vi "analysis.vi"() -> ()   [LabVIEW 2015]
doc: "Program analyzes data files for both constant radioactive decay counting and shor-lived decay experiments."
uses:
  <vilib>/Utility/file.llb/Read Delimited Spreadsheet (DBL).vi
  <vilib>/imath/engines/lvmath2/RunTimeEngine/Managers/WorkSpace/UID Generator.vi
  <vilib>/imath/engines/lvmath2/RunTimeEngine/RunTimeType/NIMS_RunTimeType_From StrictType (excl LVString).vi
  <instcachedir>/0/NIMS_RunTimeType_From StrictType (excl LVString)_EB1C38A9BC5048DA9ABDA8F781E54D21.lvgen/NIMS_RunTimeType_From StrictType (excl LVString)_EB1C38A9BC5048DA9ABDA8F781E54D21_000.vi
  <vilib>/imath/engines/lvmath2/RunTimeEngine/LocalVariableDefStatement/MC_LocalVariableDefStatement_Display.vi
  <vilib>/imath/engines/lvmath2/RunTimeEngine/Managers/SymbolTable/Clear UID.vi
  <vilib>/imath/engines/lvmath2/RunTimeEngine/NodeEndStatement/NIMS_NodeEndStatement_Output.vi
  <instcachedir>/0/NIMS_NodeEndStatement_Output_53EC0D466D134D7ABD903AC30B43404B.lvgen/NIMS_NodeEndStatement_Output_53EC0D466D134D7ABD903AC30B43404B_001.vi
  <vilib>/imath/engines/lvmath2/RunTimeEngine/ErrorHandling/NIMS_Finalize Error.vi
  <vilib>/Analysis/NI_AALBase.lvlib
  <vilib>/Analysis/NI_AALPro.lvlib
  <vilib>/imath/engines/lvmath2/RunTimeEngine/Managers/SymbolTable/NIMS_WorkSpace.lvlib
panel:
  out "Decay Time (s)":dbl=106.21083077427976
  out "Counting Statistics":T1(graph)={"X Values"=[13.5, 14.5, 15.5, 16.5, 17.5, 18.5, 19.5, 20.5, 21.5, 22.5, 23.5, 24.5, 25.5, 26.5, 27.5, 28.5, 29.5, 30.5, 31.5, 32.5, 33.5, 34.5, 35.5], "Histogram: h(x)"=[4, 1, 4, 6, 8, 9, 10, 9, 17, 13, 12, 13, 8, 13, 15, 8, 9, 4, 4, 1, 3, 3, 6]}
  out "Decay Curve":cluster{dbl[], "Best Exponential Fit":dbl[]}[](graph)=[{[1.0, 2.0, 3.0, 4.0, 5.0, 6.0, 7.0, 8.0, 9.0, 10.0, 11.0, 12.0, 13.0, 14.0, 15.0, 16.0, 17.0, 18.0, 19.0, 20.0, 21.0, 22.0, 23.0, 24.0, 25.0, 26.0, 27.0, 28.0, 29.0, 30.0, 31.0, 32.0, 33.0, 34.0, 35.0, 36.0, 37.0, 38.0, 39.0, 40.0, 41.0, 42.0, 43.0, 44.0, 45.0, 46.0, 47.0, 48.0, 49.0, 50.0, 51.0, 52.0, 53.0, 54.0, 55.0, 56.0, 57.0, 58.0, 59.0, 60.0, 61.0, 62.0, 63.0, 64.0, 65.0, 66.0, 67.0, 68.0, 69.0, 70.0, 71.0, 72.0, 73.0, 74.0, 75.0, 76.0, 77.0, 78.0, 79.0, 80.0, 81.0, 82.0, 83.0, 84.0, 85.0, 86.0, 87.0, 88.0, 89.0, 90.0, 91.0, 92.0, 93.0, 94.0, 95.0, 96.0, 97.0, 98.0, 99.0, 100.0, 101.0, 102.0, 103.0, 104.0, 105.0, 106.0, 107.0, 108.0, 109.0, 110.0, 111.0, 112.0, 113.0, 114.0, 115.0, 116.0, 117.0, 118.0, 119.0, 120.0, 121.0, 122.0, 123.0, 124.0, 125.0, 126.0, 127.0, 128.0, 129.0, 130.0, 131.0, 132.0, 133.0, 134.0, 135.0, 136.0, 137.0, 138.0, 139.0, 140.0, 141.0, 142.0, 143.0, 144.0, 145.0, 146.0, 147.0, 148.0, 149.0, 150.0, 151.0, 152.0, 153.0, 154.0, 155.0, 156.0, 157.0, 158.0, 159.0, 160.0, 161.0, 162.0, 163.0, 164.0, 165.0, 166.0, 167.0, 168.0, 169.0, 170.0, 171.0, 172.0, 173.0, 174.0, 175.0, 176.0, 177.0, 178.0, 179.0, 180.0, 181.0, 182.0, 183.0, 184.0, 185.0, 186.0, 187.0, 188.0, 189.0, 190.0, 191.0, 192.0, 193.0, 194.0, 195.0, 196.0, 197.0, 198.0, 199.0, 200.0, 201.0, 202.0, 203.0, 204.0, 205.0, 206.0, 207.0, 208.0, 209.0, 210.0, 211.0, 212.0, 213.0, 214.0, 215.0, 216.0, 217.0, 218.0, 219.0, 220.0, 221.0, 222.0, 223.0, 224.0, 225.0, 226.0, 227.0, 228.0, 229.0, 230.0, 231.0, 232.0, 233.0, 234.0, 235.0, 236.0, 237.0, 238.0, 239.0, 240.0, 241.0, 242.0, 243.0, 244.0, 245.0, 246.0, 247.0, 248.0, 249.0, 250.0, 251.0, 252.0, 253.0, 254.0, 255.0, 256.0, 257.0, 258.0, 259.0, 260.0, 261.0, 262.0, 263.0, 264.0, 265.0, 266.0, 267.0, 268.0, 269.0, 270.0, 271.0, 272.0, 273.0, 274.0, 275.0, 276.0, 277.0, 278.0, 279.0, 280.0, 281.0, 282.0, 283.0, 284.0, 285.0, 286.0, 287.0, 288.0, 289.0, 290.0, 291.0, 292.0, 293.0, 294.0, 295.0, 296.0, 297.0, 298.0, 299.0, 300.0, 301.0, 302.0, 303.0, 304.0, 305.0, 306.0, 307.0, 308.0, 309.0, 310.0, 311.0, 312.0, 313.0, 314.0, 315.0, 316.0, 317.0, 318.0, 319.0, 320.0, 321.0, 322.0, 323.0, 324.0, 325.0, 326.0, 327.0, 328.0, 329.0, 330.0], "Best Exponential Fit"=[80.0, 70.0, 60.0, 68.0, 62.0, 64.0, 57.0, 55.0, 60.0, 67.0, 62.0, 57.0, 54.0, 53.0, 54.0, 49.0, 58.0, 50.0, 44.0, 55.0, 51.0, 60.0, 51.0, 53.0, 45.0, 56.0, 49.0, 39.0, 50.0, 48.0, 53.0, 55.0, 44.0, 45.0, 36.0, 29.0, 36.0, 53.0, 41.0, 38.0, 34.0, 42.0, 50.0, 43.0, 36.0, 42.0, 43.0, 66.0, 32.0, 38.0, 41.0, 36.0, 38.0, 33.0, 33.0, 31.0, 37.0, 34.0, 33.0, 34.0, 33.0, 39.0, 37.0, 19.0, 35.0, 42.0, 35.0, 34.0, 26.0, 32.0, 35.0, 37.0, 34.0, 23.0, 21.0, 25.0, 27.0, 27.0, 30.0, 27.0, 25.0, 34.0, 26.0, 26.0, 25.0, 30.0, 32.0, 27.0, 28.0, 21.0, 29.0, 33.0, 37.0, 27.0, 27.0, 28.0, 25.0, 17.0, 18.0, 14.0, 29.0, 27.0, 27.0, 17.0, 18.0, 25.0, 24.0, 15.0, 21.0, 27.0, 24.0, 18.0, 24.0, 21.0, 16.0, 22.0, 16.0, 19.0, 18.0, 32.0, 21.0, 17.0, 25.0, 17.0, 23.0, 23.0, 17.0, 16.0, 10.0, 17.0, 23.0, 21.0, 26.0, 13.0, 16.0, 15.0, 12.0, 22.0, 21.0, 15.0, 20.0, 17.0, 16.0, 15.0, 21.0, 15.0, 13.0, 20.0, 25.0, 15.0, 14.0, 11.0, 16.0, 20.0, 13.0, 17.0, 15.0, 26.0, 10.0, 12.0, 17.0, 20.0, 13.0, 12.0, 12.0, 13.0, 16.0, 12.0, 11.0, 10.0, 11.0, 13.0, 13.0, 23.0, 10.0, 14.0, 12.0, 6.0, 9.0, 13.0, 10.0, 17.0, 8.0, 8.0, 12.0, 9.0, 10.0, 15.0, 9.0, 14.0, 9.0, 15.0, 11.0, 11.0, 9.0, 21.0, 11.0, 12.0, 8.0, 11.0, 10.0, 9.0, 12.0, 13.0, 11.0, 11.0, 10.0, 9.0, 13.0, 8.0, 11.0, 6.0, 13.0, 8.0, 11.0, 15.0, 11.0, 9.0, 10.0, 8.0, 9.0, 4.0, 6.0, 7.0, 4.0, 5.0, 9.0, 7.0, 7.0, 12.0, 7.0, 6.0, 9.0, 7.0, 7.0, 8.0, 10.0, 6.0, 7.0, 4.0, 7.0, 3.0, 7.0, 2.0, 11.0, 6.0, 9.0, 7.0, 10.0, 13.0, 3.0, 11.0, 7.0, 6.0, 6.0, 6.0, 3.0, 6.0, 4.0, 6.0, 10.0, 9.0, 8.0, 5.0, 6.0, 7.0, 6.0, 3.0, 7.0, 6.0, 4.0, 2.0, 3.0, 3.0, 5.0, 6.0, 3.0, 5.0, 6.0, 8.0, 8.0, 11.0, 6.0, 3.0, 6.0, 4.0, 7.0, 1.0, 2.0, 1.0, 4.0, 2.0, 4.0, 1.0, 7.0, 2.0, 0.0, 4.0, 4.0, 5.0, 4.0, 1.0, 3.0, 2.0, 8.0, 3.0, 4.0, 3.0, 4.0, 7.0, 5.0, 5.0, 2.0, 4.0, 2.0, 7.0, 5.0, 3.0, 2.0, 4.0, 2.0, 3.0, 4.0, 0.0, 3.0, 3.0, 4.0, 4.0, 5.0, 5.0]}, {[1.0, 2.0, 3.0, 4.0, 5.0, 6.0, 7.0, 8.0, 9.0, 10.0, 11.0, 12.0, 13.0, 14.0, 15.0, 16.0, 17.0, 18.0, 19.0, 20.0, 21.0, 22.0, 23.0, 24.0, 25.0, 26.0, 27.0, 28.0, 29.0, 30.0, 31.0, 32.0, 33.0, 34.0, 35.0, 36.0, 37.0, 38.0, 39.0, 40.0, 41.0, 42.0, 43.0, 44.0, 45.0, 46.0, 47.0, 48.0, 49.0, 50.0, 51.0, 52.0, 53.0, 54.0, 55.0, 56.0, 57.0, 58.0, 59.0, 60.0, 61.0, 62.0, 63.0, 64.0, 65.0, 66.0, 67.0, 68.0, 69.0, 70.0, 71.0, 72.0, 73.0, 74.0, 75.0, 76.0, 77.0, 78.0, 79.0, 80.0, 81.0, 82.0, 83.0, 84.0, 85.0, 86.0, 87.0, 88.0, 89.0, 90.0, 91.0, 92.0, 93.0, 94.0, 95.0, 96.0, 97.0, 98.0, 99.0, 100.0, 101.0, 102.0, 103.0, 104.0, 105.0, 106.0, 107.0, 108.0, 109.0, 110.0, 111.0, 112.0, 113.0, 114.0, 115.0, 116.0, 117.0, 118.0, 119.0, 120.0, 121.0, 122.0, 123.0, 124.0, 125.0, 126.0, 127.0, 128.0, 129.0, 130.0, 131.0, 132.0, 133.0, 134.0, 135.0, 136.0, 137.0, 138.0, 139.0, 140.0, 141.0, 142.0, 143.0, 144.0, 145.0, 146.0, 147.0, 148.0, 149.0, 150.0, 151.0, 152.0, 153.0, 154.0, 155.0, 156.0, 157.0, 158.0, 159.0, 160.0, 161.0, 162.0, 163.0, 164.0, 165.0, 166.0, 167.0, 168.0, 169.0, 170.0, 171.0, 172.0, 173.0, 174.0, 175.0, 176.0, 177.0, 178.0, 179.0, 180.0, 181.0, 182.0, 183.0, 184.0, 185.0, 186.0, 187.0, 188.0, 189.0, 190.0, 191.0, 192.0, 193.0, 194.0, 195.0, 196.0, 197.0, 198.0, 199.0, 200.0, 201.0, 202.0, 203.0, 204.0, 205.0, 206.0, 207.0, 208.0, 209.0, 210.0, 211.0, 212.0, 213.0, 214.0, 215.0, 216.0, 217.0, 218.0, 219.0, 220.0, 221.0, 222.0, 223.0, 224.0, 225.0, 226.0, 227.0, 228.0, 229.0, 230.0, 231.0, 232.0, 233.0, 234.0, 235.0, 236.0, 237.0, 238.0, 239.0, 240.0, 241.0, 242.0, 243.0, 244.0, 245.0, 246.0, 247.0, 248.0, 249.0, 250.0, 251.0, 252.0, 253.0, 254.0, 255.0, 256.0, 257.0, 258.0, 259.0, 260.0, 261.0, 262.0, 263.0, 264.0, 265.0, 266.0, 267.0, 268.0, 269.0, 270.0, 271.0, 272.0, 273.0, 274.0, 275.0, 276.0, 277.0, 278.0, 279.0, 280.0, 281.0, 282.0, 283.0, 284.0, 285.0, 286.0, 287.0, 288.0, 289.0, 290.0, 291.0, 292.0, 293.0, 294.0, 295.0, 296.0, 297.0, 298.0, 299.0, 300.0, 301.0, 302.0, 303.0, 304.0, 305.0, 306.0, 307.0, 308.0, 309.0, 310.0, 311.0, 312.0, 313.0, 314.0, 315.0, 316.0, 317.0, 318.0, 319.0, 320.0, 321.0, 322.0, 323.0, 324.0, 325.0, 326.0, 327.0, 328.0, 329.0, 330.0], "Best Exponential Fit"=[62.77238848490245, 62.184145225125434, 61.60141442299143, 61.024144420978196, 60.4522840456488, 59.885782603115175, 59.324589874544294, 58.768656111706356, 58.217932032564796, 57.6723688169075, 57.13191810201907, 56.59653197839359, 56.06616298548755, 55.54076410751265, 55.02028876926792, 54.504690832010986, 53.99392458936799, 53.48794476328183, 52.98670649999839, 52.490165366090395, 51.99827734451846, 51.51099883072915, 51.02828662878951, 50.55009794755788, 50.07639039689059, 49.60712198388416, 49.14225110915277, 48.681736563140525, 48.22553752246845, 47.773613546315495, 47.325924572833614, 46.882430915596395, 46.443093260080964, 46.007872660182834, 45.57673053476346, 45.149628664230114, 44.72652918714783, 44.30739459688307, 43.89218773827891, 43.48087180436125, 43.07341033307606, 42.669767204057074, 42.269906635423816, 41.87379318060965, 41.481391725219524, 41.092667483917175, 40.707585997341496, 40.326113129051826, 39.94821506250183, 39.57385829804175, 39.20300964994877, 38.83563624348516, 38.471705511984055, 38.11118519396249, 37.754043330261474, 37.40024826121297, 37.04976862383329, 36.70257334904286, 36.35863165891203, 36.01791306393274, 35.680387360315635, 35.34602462731263, 35.01479522456449, 34.686669789473285, 34.36161923459953, 34.03961474508359, 33.72062777609137, 33.40463005028385, 33.091593555310425, 32.781490541325645, 32.47429351852928, 32.16997525472944, 31.868508772928458, 31.569867348931524, 31.274024508977618, 30.98095402739268, 30.690629924264783, 30.403026463141085, 30.118118148746355, 29.835879724722886, 29.556286171391598, 29.2793127035341, 29.004934768195547, 28.733128042508078, 28.46386843153469, 28.197132066133253, 27.93289530084059, 27.67113471177636, 27.411827094566625, 27.15494946228679, 26.900479043423925, 26.648393279858105, 26.398669824862704, 26.151286541123405, 25.906221498775796, 25.66345297346135, 25.422959444401613, 25.184719592490442, 24.948712298404136, 24.714916640729236, 24.483311894107935, 24.253877527400807, 24.026593201866785, 23.801438769360182, 23.578394270544614, 23.357439933123654, 23.13855617008808, 22.921723577979527, 22.70692293517045, 22.494135200160134, 22.283341509886753, 22.074523178055188, 21.867661693480564, 21.662738718447233, 21.459736087083257, 21.258635803749982, 21.059420041446817, 20.862071140230903, 20.666571605651605, 20.47290410719968, 20.28105147677097, 20.090996707144505, 19.90272295047485, 19.716213516798575, 19.53145187255478, 19.348421639119376, 19.16710659135322, 18.987490656163775, 18.80955791108026, 18.6332925828422, 18.45867904600114, 18.2857018215355, 18.114345575478403, 17.94459511755837, 17.776435399852712, 17.609851515453606, 17.444828697146615, 17.281352316101643, 17.119407880576084, 16.958981034630206, 16.80005755685451, 16.642623359109077, 16.486664485274638, 16.332167110015448, 16.17911753755368, 16.027502200455345, 15.877307658427576, 15.728520597127172, 15.581127826980323, 15.43511628201339, 15.290473018694636, 15.147185214786829, 15.005240168210571, 14.864625295918305, 14.72532813277885, 14.587336330472406, 14.450637656395914, 14.315219992578655, 14.181071334608044, 14.04817979056545, 13.916533579972027, 13.786121032744386, 13.656930588160105, 13.528950793832857, 13.40217030469724, 13.27657788200302, 13.152162392318871, 13.028912806545422, 12.906818198937554, 12.785867746135867, 12.666050726207216, 12.547356517694231, 12.429774598673767, 12.313294545824164, 12.19790603350123, 12.083598832822922, 11.970362810762571, 11.858187929250615, 11.747064244284756, 11.636981905048453, 11.527931153037667, 11.4199023211958, 11.312885833056736, 11.20687220189591, 11.10185202988934, 10.997816007280534, 10.8947549115552, 10.7926596066237, 10.691521042011153, 10.591330252055158, 10.492078355110973, 10.393756552764218, 10.296356129050896, 10.19986844968476, 10.10428496129189, 10.009597190652483, 9.915796743949704, 9.822875306025608, 9.730824639644014, 9.639636584760307, 9.549303057798067, 9.45981605093248, 9.37116763138047, 9.283349940697473, 9.196355194080812, 9.110175679679598, 9.024803757911082, 8.940231860783443, 8.856452491224893, 8.773458222419087, 8.691241697146761, 8.609795627133526, 8.529112792403774, 8.449186040640681, 8.370008286552128, 8.29157251124263, 8.213871761591154, 8.13689914963469, 8.060647851957702, 7.985111109087217, 7.91028222489364, 7.836154565997136, 7.7627215611796245, 7.689976700802231, 7.617913536228255, 7.546525679251489, 7.475806801529931, 7.405750634024808, 7.3363509664448125, 7.267601646695612, 7.199496580334447, 7.132029730029907, 7.065195115026712, 6.9989868106155555, 6.9333989476078735, 6.868425711815573, 6.804061343535621, 6.7403001370394415, 6.677136440067148, 6.614564653326458, 6.552579229996354, 6.491174675235348, 6.430345545694408, 6.370086449034391, 6.310392043448046, 6.251257037186472, 6.192676188090009, 6.1346443031235545, 6.077156237916191, 6.0202068963051785, 5.963791229884162, 5.907904237555675, 5.85254096508778, 5.797696504674907, 5.743365994502779, 5.689544618317432, 5.63622760499826, 5.583410228135074, 5.531087805609119, 5.479255699178009, 5.427909314064571, 5.377044098549515, 5.326655543567953, 5.276739182309668, 5.227290589823157, 5.178305382623357, 5.129779218303072, 5.081707795148023, 5.034086851755512, 4.9869121666566745, 4.940179557942233, 4.893884882891808, 4.848024037606652, 4.802592956645875, 4.757587612666029, 4.713004016064118, 4.668838214623911, 4.625086293165603, 4.581744373198738, 4.538808612578386, 4.496275205164565, 4.454140380484813, 4.41240040339997, 4.371051573773043, 4.330090226141225, 4.289512729390936, 4.249315486435959, 4.2094949338985455, 4.170047541793545, 4.130969813215484, 4.092258284028557, 4.053909522559566, 4.0159201292936855, 3.978286736573127, 3.9410060082985883, 3.904074639633528, 3.8674893567111934, 3.8312469163444103, 3.795344105738071, 3.759777742204336, 3.7245446728805005, 3.689641774449492, 3.655065952863006, 3.6208141430672187, 3.586883308731087, 3.5532704419771757, 3.5199725631150285, 3.4869867203770153, 3.454309989656676, 3.4219394742494984, 3.3898723045961345, 3.35810563802803, 3.326636658515417, 3.2954625764176897, 3.264580628236104, 3.2339880763688074, 3.2036822088681505, 3.1736603392002882, 3.1439198060070157, 3.114457972869858, 3.085272228076348, 3.0563599843885094, 3.0277186788135095, 2.999345772376448, 2.9712387498952904, 2.9433951197579002, 2.915812413701168, 2.8884881865921987, 2.86142001621157, 2.834605503038595]}]
  in  "Constant-File Path":path=path "C:/Users/mylicon/Desktop/week8/sample-constant.txt" caption="Select data file for Histogram Plot with Poisson overlay:"
  in  "Decay-File Path":path=path "C:/Users/mylicon/Desktop/week8/sample-countratedata.txt" caption="Select data file for decay plot with exponential overlay:"
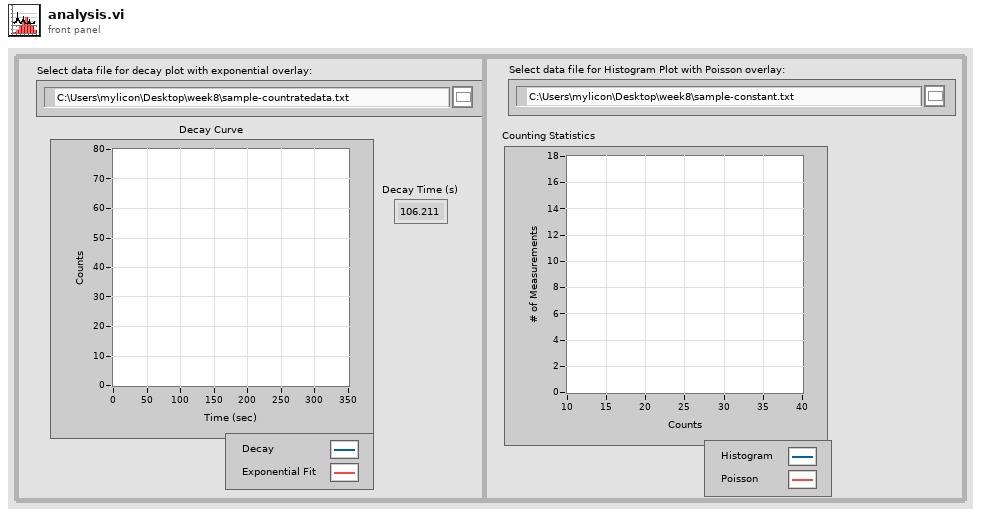
[diagram p1: front panel]
types:
  T1 = cluster{"X Values":dbl[], "Histogram: h(x)":i32[]}
  T2 = cluster{"all rows":dbl[], "Best Exponential Fit":dbl[]}
  T3 = cluster{"all rows":dbl[], "Best Exponential Fit":dbl[]}[]
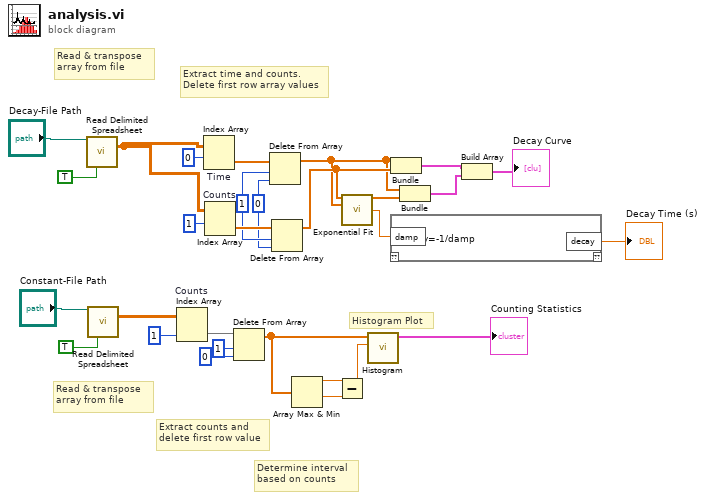
[diagram p0: block diagram]
diagram:
  w15 = 0 ("index")
  w20 = 1 ("length")
  # "Histogram Plot"
  # "Determine interval \nbased on counts"
  # "Extract counts and\ndelete first row value"
  # "Read & transpose \narray from file"
  # "Extract time and counts.\nDelete first row array values"
  # "Read & transpose \narray from file"
  n1 = call-poly <vilib>:"Read Delimited Spreadsheet.vi"("file path (dialog if empty)"="Decay-File Path", "transpose? (F)"=TRUE) -> ("all rows"=w4:dbl[][])  [unwired: 8 in, 5 out]
  n2 = call-poly <vilib>:"Read Delimited Spreadsheet.vi"("file path (dialog if empty)"="Constant-File Path", "transpose? (F)"=TRUE) -> ("all rows"=w12:dbl[][])  [unwired: 8 in, 5 out]
  n3 = Index Array "Counts"(array=w12, index (row)=1) -> (element=w24:dbl[])  [unwired: 1 in]
  n4 = Index Array "Time"(array=w4, index (row)=0) -> (element=w22:dbl[])  [unwired: 1 in]
  n5 = Index Array "Counts"(array=w4, index (row)=1) -> (element=w21:dbl[])  [unwired: 1 in]
  n6 = Delete From Array(array=w24, length=1, index=0) -> (array with subset deleted=w14:dbl[])  [unwired: 1 out]
  n7 = Delete From Array(array=w22, length=w20, index=w15) -> (array with subset deleted=w9:dbl[])  [unwired: 1 out]
  n8 = Delete From Array(array=w21, length=w20, index=w15) -> (array with subset deleted=w11:dbl[])  [unwired: 1 out]
  n9 = Array Max & Min(array=w14) -> (max value=w19:dbl, min value=w18:dbl)  [unwired: 2 out]
  n10 = Subtract(x=w19, y=w18) -> (x-y=w17:dbl)
  n11 = call <vilib>:"Exponential Fit.vi"("Y"=w11, "X"=w9) -> ("Best Exponential Fit"=w10:dbl[], "damping"=w3:dbl)  [unwired: 8 in, 4 out]
  n12 = call <vilib>:"Histogram.vi"("intervals"=w17, "X"=w14) -> ("Histogram Graph"=→"Counting Statistics":T1)  [unwired: 6 in, 3 out]
  n13 = Bundle("all rows"=w9, "all rows"=w11) -> (w8:cluster{"all rows":dbl[], "all rows":dbl[]})  [unwired: 1 in]
  n14 = mathscript code="decay=-1/damp"("damp"=w3) -> ("decay"=→"Decay Time (s)":dbl)  [unwired: 1 in, 1 out]
  n15 = Bundle("all rows"=w9, "Best Exponential Fit"=w10) -> (w7:T2)  [unwired: 1 in]
  n16 = Build Array(w8, w7) -> (→"Decay Curve":T3)
